vi "day_2.vi"() -> ()   [LabVIEW 2020]
panel:
  out "output 3":string
  out "output 2":string
  out "output 1":string
  in  "delay_time":u32
  in  "Logging Button":bool
  out "Loop Count":i32
  out "appended array":cluster{i32, i32, i32}[](array[cluster])
  out "Numeric":i32
  out "cluster":cluster{i32, i32, i32}
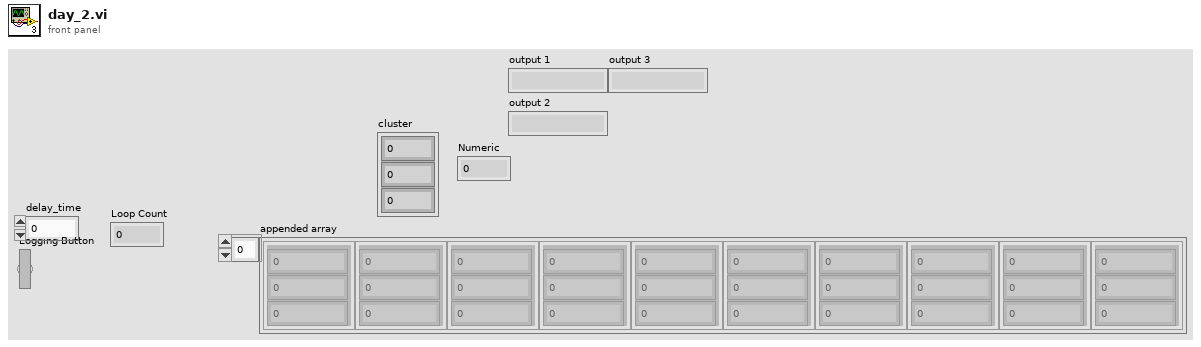
[diagram p1: front panel]
types:
  T1 = enum16{"open", "replace", "create", "open or create", "replace or create", "replace or create with confirmation"}
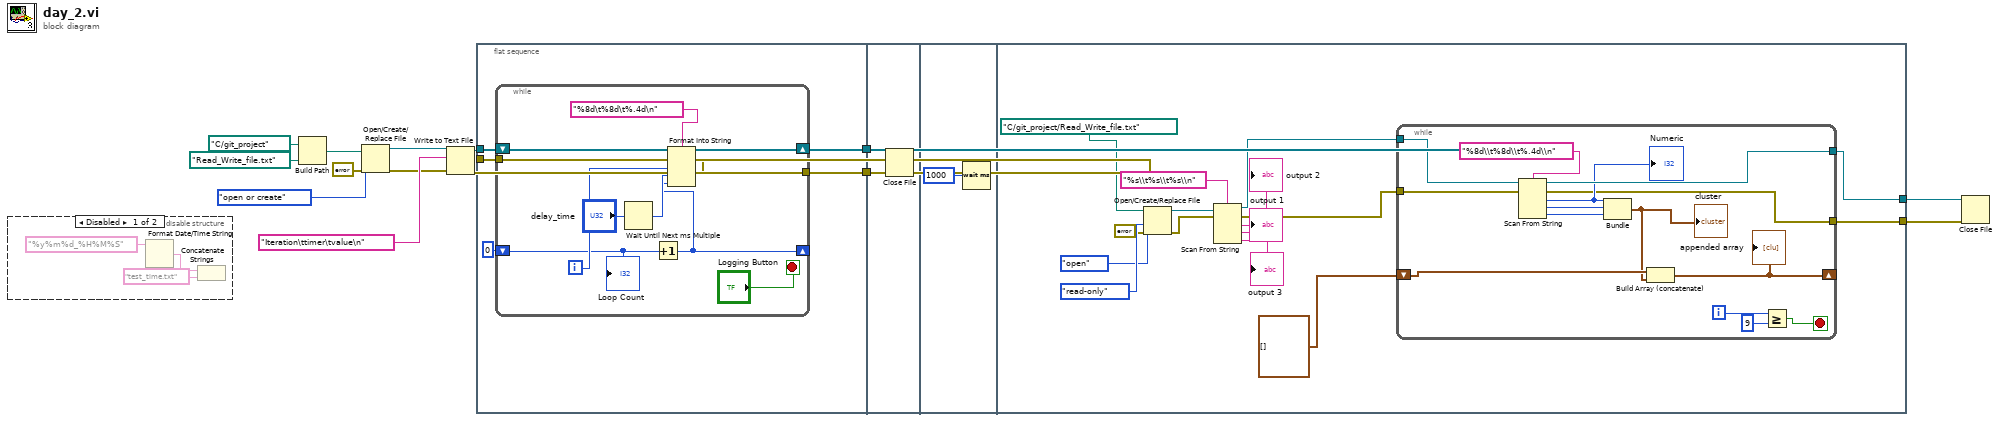
[diagram p0: block diagram]
diagram:
  n1 = disable-structure shown="Disabled" {
    frame Disabled {
      n2 = Format Date/Time String(time format string (%c)="%y%m%d_%H%M%S") -> (date/time string=w16:string)  [unwired: 2 in]
      n3 = Concatenate Strings(w16, "test_time.txt" ("string")) -> ()  [unwired: 1 out]
    }
    frame Enabled {
    }
  }
  n4 = Build Path(base path=path "C:/git_project", name or relative path=path "Read_Write_file.txt") -> (appended path=w13:path)
  n5 = Open/Create/Replace File(file path (use dialog)=w13, error in=errorcluster {"status"=FALSE, "code"=0, "source"=""}, operation (0:open)=T1."open or create") -> (refnum out=w11:refnum<file>, error out=w7:errorcluster)  [unwired: 3 in, 1 out]
  n6 = Write to Text File(file (use dialog)=w11, text="Iteration\ttimer\tvalue\n", error in=w7) -> (refnum out=w9:refnum<file>, error out=w6:errorcluster)  [unwired: 1 in, 1 out]
  n7 = flat-sequence {
    tunnel: w9 -> [w22]
    tunnel: w6 -> [w20]
    tunnel: [w19] -> w5
    tunnel: [w18] -> w4
    tunnel: w5 -> [w35]
    tunnel: w4 -> [w34]
    tunnel: [w44] -> w2
    tunnel: [w40] -> w1
    frame #0 {
      n8 = while {
        shift-right: [w32] -> w18
        shift-left: w22 -> [w33]
        shift-right: [w27] -> _
        shift-left: 0 -> [w28]
        tunnel: w20 -> [w24]
        tunnel: [w23] -> w19
        i -> [w31]
        stop <- "Logging Button" stop-if-true
        n9 = Wait Until Next ms Multiple(millisecond multiple="delay_time") -> (millisecond timer value=w29:u32)
        n10 = Increment(x=w28) -> (x+1=w27:i32)
        n11 = Format Into String(format string="%8d\t%8d\t%.4d\n", initial string=w33, error in=w24, w31, w29, w27) -> (resulting string=w32:refnum<file>, error out=w23:errorcluster)
        "Loop Count" <- w28
      }
    }
    frame #1 {
      n12 = Close File(refnum=w34, error in=w35) -> ()  [unwired: 2 out]
    }
    frame #2 {
      n13 = Wait (ms)(milliseconds to wait=u32 1000) -> ()  [unwired: 1 out]
    }
    frame #3 {
      n14 = Open/Create/Replace File(file path (use dialog)=path "C:/git_project/Read_Write_file.txt" ("name or relative path"), error in=errorcluster {"status"=FALSE, "code"=0, "source"=""}, operation (0:open)=T1."open", access (0:read/write)=enum16{"read/write", "read-only", "write-only"}."read-only") -> (refnum out=w50:refnum<file>, error out=w42:errorcluster)  [unwired: 2 in, 1 out]
      n15 = Scan From String("%s\\t%s\\t%s\\n" ("format string"), w50, w42) -> (w51:refnum<file>, w41:errorcluster, output 1=→"output 1":string, output 2=→"output 2":string, output 3=→"output 3":string)  [unwired: 3 in]
      n16 = while {
        tunnel: w51 -> [w65]
        tunnel: [w63] -> w44
        shift-right: [w60] -> _
        shift-left: cluster{i32, i32, i32}[] [] ("Array") -> [w55]
        tunnel: w41 -> [w53]
        tunnel: [w52] -> w40
        i -> [w58]
        stop <- w59 stop-if-true
        n17 = Scan From String("%8d\\t%8d\\t%.4d\\n" ("format string"), w65, w53) -> (w63:refnum<file>, w52:errorcluster, output 1=w56:i32, output 2=w62:i32, output 3=w61:i32)  [unwired: 3 in]
        "Numeric" <- w56
        n18 = Bundle("Numeric"=w56, w62, w61) -> (w54:cluster{"Numeric":i32, i32, i32})  [unwired: 1 in]
        "cluster" <- w54
        n19 = Build Array (concatenate)(w55, w54) -> (w60:cluster{"Numeric":i32, i32, i32}[])
        "appended array" <- w60
        n20 = Greater Or Equal?(x=w58, y=9) -> (x >= y?=w59:bool)
      }
    }
  }
  n21 = Close File(refnum=w2, error in=w1) -> ()  [unwired: 2 out]
